vi "Spectrum.vi"(2 "Gain":dbl=1.0, 3 "Remove Polynomial Order":i32=2, 4 "Waveform 1":cluster{dbl, dbl, dbl[]}, 5 "Binning":bool) -> (1 "Cluster":T1)   [LabVIEW 2010]
uses:
  <vilib>/measure/NI_MAPro.lvlib
  <vilib>/measure/maspectr.llb/FFT Power Spectrum and PSD for 1 Chan.vi
  <vilib>/Analysis/4window.llb/windowTd.ctl
  <vilib>/Analysis/NI_AALPro.lvlib
  <vilib>/measure/maspectr.llb/Power Spectrum and PSD Export Mode.ctl
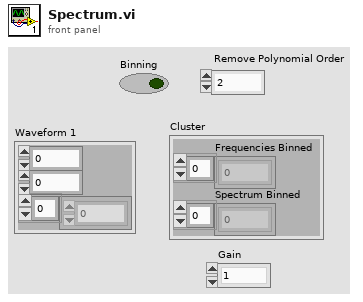
[diagram p1: front panel]
types:
  T1 = cluster{"Frequencies Binned":dbl[], "Spectrum Binned":dbl[]}
  T2 = typedef "NI_MAPro.lvlib/Power Spectrum and PSD Export Mode.ctl" = u16
  T3 = typedef "NI_AALPro.lvlib/windowTd.ctl" = u32
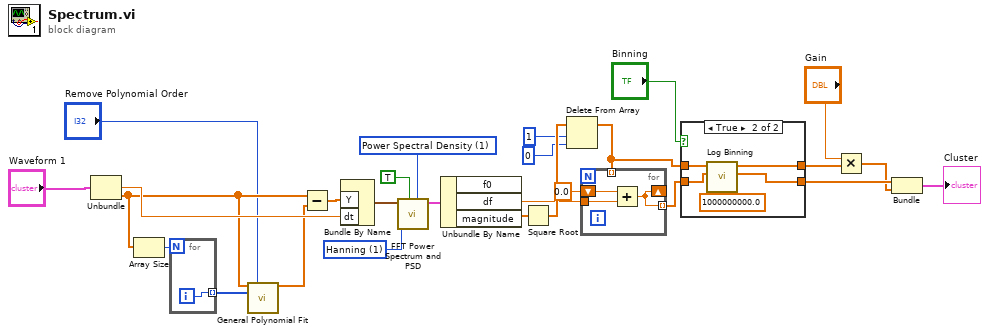
[diagram p0: block diagram]
diagram:
  w19 = T2 1 items=["Power Spectrum", "Power Spectral Density"] ("export mode")
  w16 = T3 1 items=["Rectangle"=0, "Hanning"=1, "Hamming"=2, "Blackman-Harris"=3, "Exact Blackman"=4, "Blackman"=5, "Flat Top"=6, "4 Term B-Harris "=7, "7 Term B-Harris"=8, "Low Sidelobe"=9, "Blackman Nuttall"=11, "Triangle"=30, "Bartlett-Hanning"=31, "Bohman"=32, "Parzen"=33, "Welch"=34, "Kaiser"=60, "Dolph-Chebyshev"=61, "Gaussian"=62] ("window")
  n1 = Unbundle("Waveform 1") -> (w9:dbl, w6:dbl[])  [unwired: 1 out]
  n2 = Array Size(array=w6) -> (size(s)=w8:i32)
  n3 = for {
    N: w8 -> [_]
    tunnel: [w28] -> w7 mode=indexing
    i -> [w28]
  }
  n4 = call <vilib>:"General Polynomial Fit.vi"("Y"=w6, "polynomial order"="Remove Polynomial Order", "X"=w7) -> ("Best Polynomial Fit"=w5:dbl[])  [unwired: 9 in, 3 out]
  n5 = Subtract(x=w6, y=w5) -> (x-y=w13:dbl[])
  n6 = Bundle By Name("Y"=w13, "dt"=w9) -> (w21:waveform(dbl))  [unwired: 1 in]
  n7 = call-poly <vilib>:"FFT Power Spectrum and PSD.vi"("export mode"=w19, "restart averaging (F)"=TRUE, "window"=w16, "time signal"=w21) -> ("Power Spectrum / PSD"=w14:cluster{"f0":dbl, "df":dbl, "magnitude":dbl[]})  [unwired: 4 in, 3 out]
  n8 = Unbundle By Name(w14) -> ("df"=w15:dbl, "magnitude"=w20:dbl[])  [unwired: 1 out]
  n9 = Square Root(x=w20) -> (sqrt(x)=w25:dbl[])
  n10 = Delete From Array(array=w25, length=1, index=0) -> (array with subset deleted=w26:dbl[])  [unwired: 1 out]
  n11 = for {
    tunnel: w15 -> [w31]
    shift-right: [w29] -> _
    shift-left: 0.0 -> [w30]
    tunnel: [w29] -> w18 mode=indexing
    tunnel: w26 -> [_] mode=indexing
    n12 = Add(x=w30, y=w31) -> (x+y=w29:dbl)
  }
  n13 = case shown="True" "Binning" {
    tunnel: [w32 w38] -> w12
    tunnel: w18 -> [w32 w37]
    tunnel: [w33 w36] -> w3
    tunnel: w26 -> [w33 w35]
    frame False {
    }
    frame True {
      n14 = call "Log Binning.vi"("Max Freq"=dbl[unit] 1000000000.0, "Frequencies"=w37, "Spectrum"=w35) -> ("Frequencies Binned"=w38:dbl[], "Spectrum Binned"=w36:dbl[])  [unwired: 3 in]
    }
  }
  n15 = Multiply(x="Gain", y=w3) -> (x*y=w2:dbl[])
  n16 = Bundle("Frequencies Binned"=w12, w2) -> (→"Cluster":cluster{"Frequencies Binned":dbl[], dbl[]})  [unwired: 1 out]
